vi "get plugin value by id.vi"(8 "error in (no error)":errorcluster, 10 "id":string, 11 "configuration file cluster in":T3) -> (0 "error out":errorcluster, 1 "found?":bool, 2 "plugin":T1, 3 "configuration file cluster out":T3)   [LabVIEW 2017, in "DSF Configuration API v1.0.0.lvlib"]
uses:
  DSF Configuration API v1.0.0.lvlib
  Controls/dsf configuration file/1.0.0/dsf configuration.ctl
  Controls/dsf configuration file/1.0.0/version.ctl
  Controls/dsf configuration file/1.0.0/dsf plugin.ctl
  Controls/dsf configuration file/1.0.0/dsf timing.ctl
  Controls/dsf configuration file/1.0.0/dsf group.ctl
  Controls/dsf configuration file/1.0.0/dsf transfer.ctl
  Controls/dsf configuration file/1.0.0/dsf channel.ctl
  Controls/dsf configuration file/1.0.0/dsf settings.ctl
  get item index by id/get plugin index by id.vi
  Controls/dsf configuration file/1.0.0/dsf configuration file v1.0.0.lvlib
panel:
  # "dsf file"
  # "dsf file"
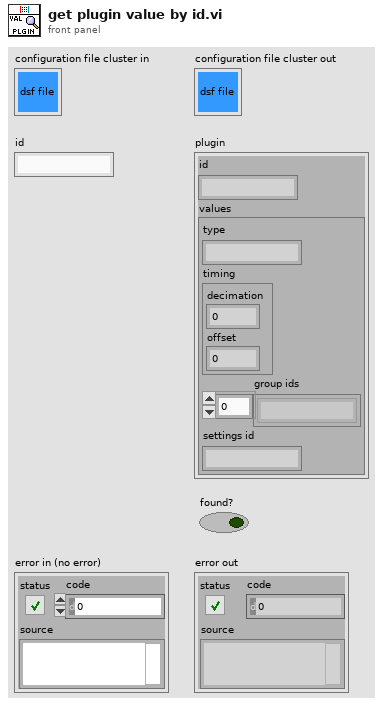
[diagram p1: front panel]
types:
  T1 = typedef "dsf configuration file v1.0.0.lvlib/dsf plugin.ctl" = cluster{"id":string, "values":cluster{"type":string, "timing":T2, "group ids":string[], "settings id":string}}
  T2 = typedef "dsf configuration file v1.0.0.lvlib/dsf timing.ctl" = cluster{"decimation":i32, "offset":i32}
  T3 = typedef "dsf configuration file v1.0.0.lvlib/dsf configuration.ctl" = cluster{"dsf":T4, "configuration":T4, "plugins":T1[], "groups":T5[], "transfers":T6[], "channels":T7[], "settings":T8[]}
  T4 = typedef "dsf configuration file v1.0.0.lvlib/version.ctl" = cluster{"major":u32, "minor":u32, "fix":u32, "build":string}
  T5 = typedef "dsf configuration file v1.0.0.lvlib/dsf group.ctl" = cluster{"id":string, "values":cluster{"direction":i32, "timing":T2, "transfer ids":string[], "settings id":string}}
  T6 = typedef "dsf configuration file v1.0.0.lvlib/dsf transfer.ctl" = cluster{"id":string, "values":cluster{"byte order":i32, "channel ids":string[], "settings id":string}}
  T7 = typedef "dsf configuration file v1.0.0.lvlib/dsf channel.ctl" = cluster{"id":string, "values":cluster{"count":i32, "offset":i32, "data type":i32, "resource path":string, "settings":string}}
  T8 = typedef "dsf configuration file v1.0.0.lvlib/dsf settings.ctl" = cluster{"id":string, "values":cluster{"key":string, "value":string}[]}
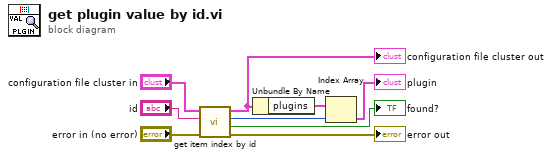
[diagram p0: block diagram]
diagram:
  n1 = call-poly "get item index by id.vi"("error in (no error)"="error in (no error)", "id"="id", "configuration file cluster in"="configuration file cluster in") -> ("error out"=→"error out":errorcluster, "found?"=→"found?":bool, "index"=w5:i32, "configuration file cluster out"=w7:T3)  [unwired: 5 in]
  "configuration file cluster out" <- w7
  n2 = Unbundle By Name(w7) -> ("plugins"=w6:T1[])
  n3 = Index Array(array=w6, index=w5) -> (element=→"plugin":T1)
